vi "Set Timeout Trigger.vi"(8 "error in (no error)":errorcluster, 10 "Trigger Settings":T1, 11 "Oscilloscope in":refnum<class "Oscilloscope.lvclass">) -> (0 "error out":errorcluster, 3 "Oscilloscope out":refnum<class "Oscilloscope.lvclass">)   [LabVIEW 2018, in "Oscilloscope.lvlib" / "Oscilloscope.lvclass"]
doc: "This Override is used to configure a TimeOut Trigger."
uses:
  Oscilloscope.lvclass
  Custom Controls/Timeout Trigger Settings.ctl
  Custom Controls/Analog Channels.ctl
  Custom Controls/Trigger Mode.ctl
  Custom Controls/Trigger Polarity.ctl
  Oscilloscope.lvlib
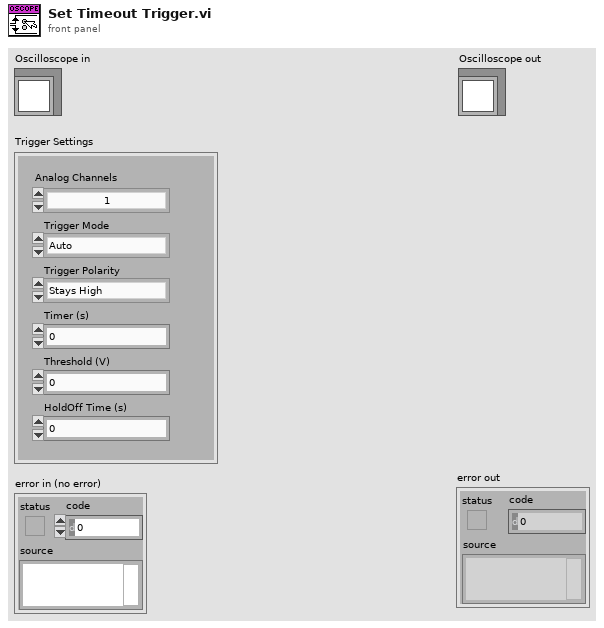
[diagram p1: front panel]
types:
  T1 = typedef "Oscilloscope.lvlib/Timeout Trigger Settings.ctl" = cluster{"Analog Channels":T2, "Trigger Mode":T3, "Trigger Polarity":T4, "Timer (s)":dbl, "Threshold (V)":dbl, "HoldOff Time (s)":dbl}
  T2 = typedef "Oscilloscope.lvlib/Analog Channels.ctl" = enum16{"1", "2", "3", "4", "5", "6", "7", "8", "9", "10", "11", "12", "13", "14", "15", "16"}
  T3 = typedef "Oscilloscope.lvlib/Trigger Mode.ctl" = enum16{"Auto", "Normal"}
  T4 = typedef "Oscilloscope.lvlib/Trigger Polarity.ctl" = enum16{"Stays High", "Stays Low", "Either"}
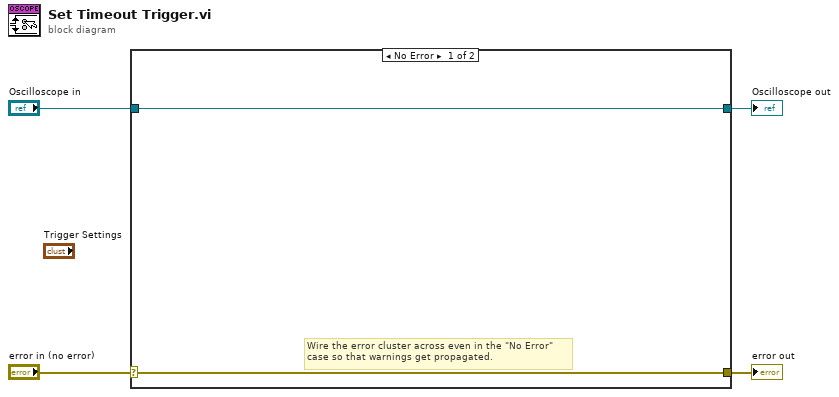
[diagram p0: block diagram]
diagram:
  n1 = case shown="No Error" "error in (no error)" {
    selector: "error in (no error)" -> [w5 w8]
    tunnel: [w5 w8] -> w3
    tunnel: [w6 w7] -> w1
    tunnel: "Oscilloscope in" -> [w6 w7]
    frame No Error {
      # "Wire the error cluster across even in the \"No Error\"\ncase so that warnings get propagated."
    }
    frame Error {
    }
  }
  "error out" <- w3
  "Oscilloscope out" <- w1
